vi "HexStringToBigInt.vi"(1 "String (hex)":string) -> (0 "Int":cluster{"P/N":bool, "Array":u64[]})   [LabVIEW 2023]
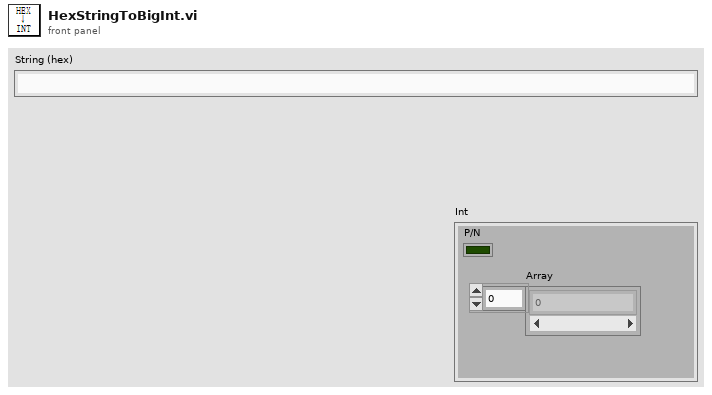
[diagram p1: front panel]
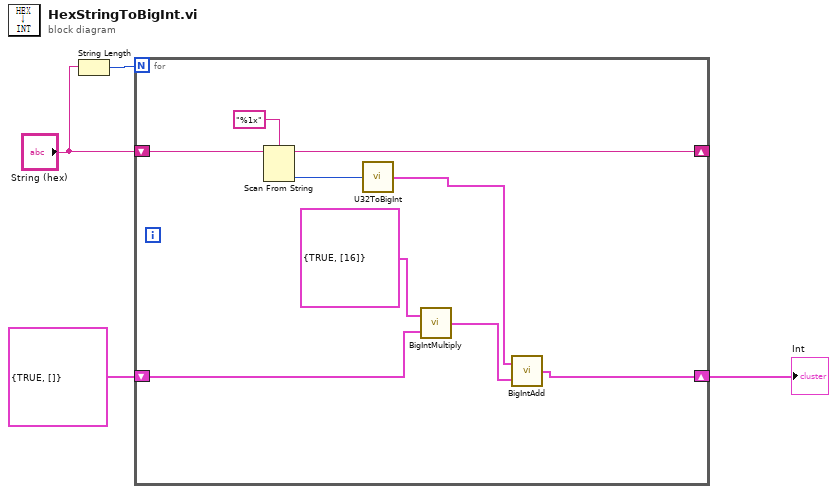
[diagram p0: block diagram]
diagram:
  n1 = String Length(string="String (hex)") -> (length=w2:i32)
  n2 = for {
    N: w2 -> [_]
    shift-right: [w10] -> w1
    shift-left: cluster{bool, u64[]} {TRUE, []} -> [w8]
    shift-right: [w9] -> _
    shift-left: "String (hex)" -> [w13]
    n3 = Scan From String(format string="%1x", input string=w13) -> (remaining string=w9:string, output 1=w11:u32)  [unwired: 3 in, 2 out]
    n4 = call "U32ToBigInt.vi"("U32 (<1e9)"=w11) -> ("Big Number"=w7:cluster{"P/N":bool, "Array":dbl[]})
    n5 = call "BigIntMultiply.vi"("b"=w8, "a"=cluster{bool, u64[]} {TRUE, [16]}) -> ("a * b"=w5:cluster{"Boolean":bool, "Array":u64[]})
    n6 = call "BigIntAdd.vi"("b"=w5, "a"=w7) -> ("a + b"=w10:cluster{"Boolean":bool, "Array":u64[]})
  }
  "Int" <- w1
